vi "R vs T measurement - SImple.vi"() -> ()   [LabVIEW 2017]
uses:
  <vilib>/Utility/file.llb/Write Delimited Spreadsheet (DBL).vi
panel:
  in  "Tab Control":enum32{"Controlls"}(tab)
  in  "Source Meter address":refnum<visa-resource-name>="GPIB1::29::INSTR"
  out "Measured Resistance (Ohms)":dbl format="%#_6p"
  in  "Resistance Range Lower Limit (2 Ohm)":dbl=2.0 format="%#_6p"
  in  "Resistance Range Upper Limit (2E+8 Ohm)":dbl=200000000.0 format="%#_6p"
  in  "Resistance NPLC (0.1)":dbl=0.1
  in  "Resistance Range (2 Ohm)":dbl=2.0
  in  "Resistance Auto Range (T: Enable)":bool=TRUE
  in  "file to save data (dialog if empty)":path
  in  "Temperature controller Addres":refnum<visa-resource-name>
  in  "Input (0:A)":u16(ring) items=["A", "B", "C", "D"]
  out "Measured Temp (K)":dbl format="%.6p"
  in  "Record Rate (ms)":u32=1000
  in  "stop":bool
  in  "Error In":errorcluster
  # "Resistance vs Temperature Measurement"
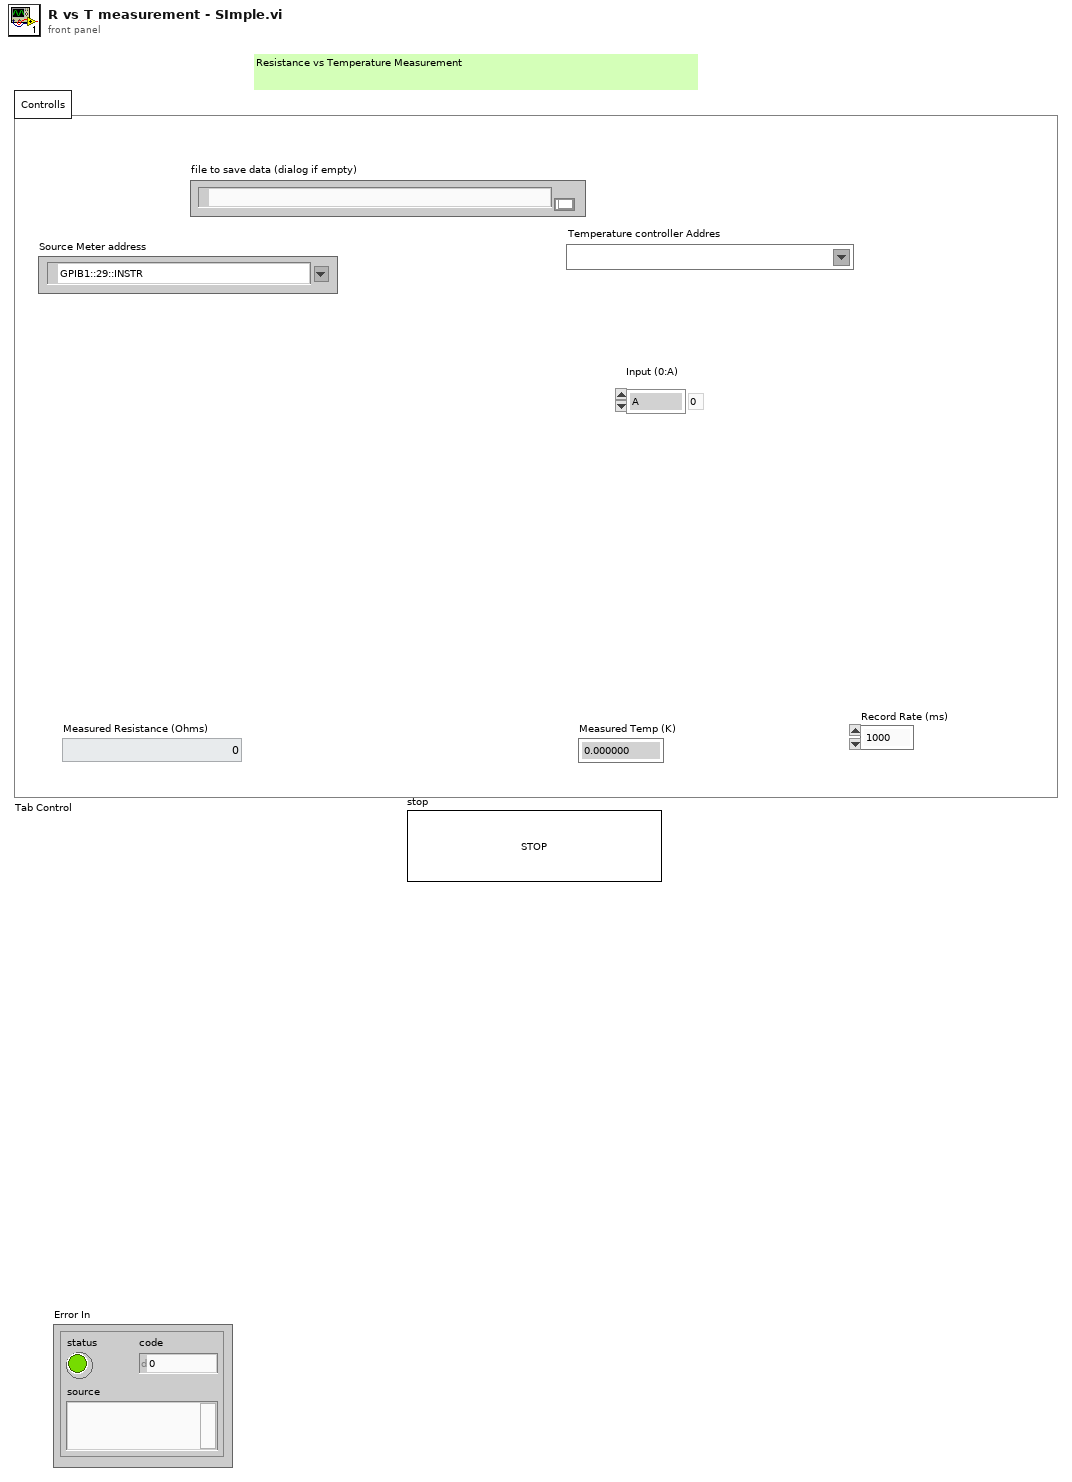
[diagram p1: front panel]
types:
  T1 = cluster{"Baud Rate":u32, "Parity":u16, "Data Bits":u16, "Stop Bits":u16, "Flow Control":u16}
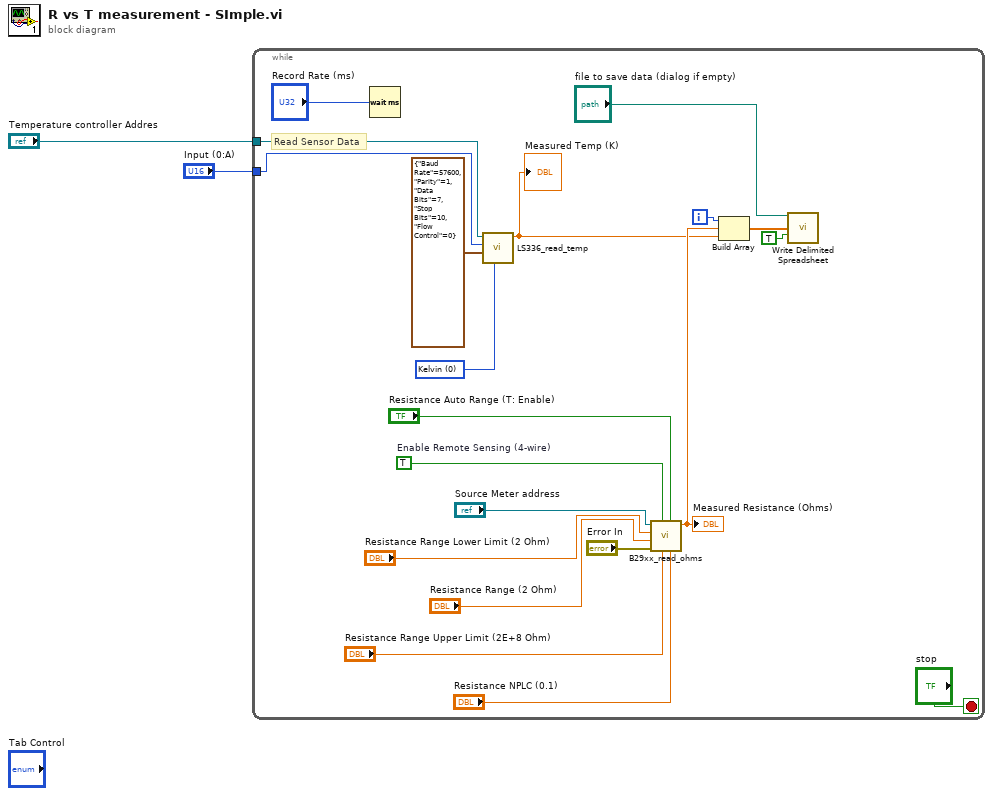
[diagram p0: block diagram]
diagram:
  n1 = while {
    tunnel: "Temperature controller Addres" -> [w9]
    tunnel: "Input (0:A)" -> [w8]
    i -> [w4]
    stop <- "stop" stop-if-true
    w10 = u16 0 items=["Kelvin", "Celsius", "Sensor Units"] ("Data Source (0:Kelvin)")
    w20 = TRUE  # Enable Remote Sensing (4-wire)
    # "Read Sensor Data"
    n2 = Wait (ms)(milliseconds to wait="Record Rate (ms)") -> ()  [unwired: 1 out]
    n3 = call "LS336_read_temp.vi"("Data Source (0:Kelvin)"=w10, "Serial Configuration"=T1 {"Baud Rate"=57600, "Parity"=1, "Data Bits"=7, "Stop Bits"=10, "Flow Control"=0}, "Input (0:A)"=w8, "VISA Refnum in"=w9) -> ("Sensor Data"=w3:dbl)  [unwired: 7 in]
    "Measured Temp (K)" <- w3
    n4 = call "B29xx_read_ohms.vi"("Resistance NPLC (0.1)"="Resistance NPLC (0.1)", "Resistance Auto Range (T: Enable)"="Resistance Auto Range (T: Enable)", "Resistance Range Upper Limit (2E+8 Ohm)"="Resistance Range Upper Limit (2E+8 Ohm)", "Enable Remote Sensing (4-wire)"=w20, "error in (no error)"="Error In", "Resistance Range (2 Ohm)"="Resistance Range (2 Ohm)", "Resistance Range Lower Limit (2 Ohm)"="Resistance Range Lower Limit (2 Ohm)", "VISA Refnum in"="Source Meter address") -> ("Measurement Result"=w14:dbl)  [unwired: 2 in, 1 out]
    "Measured Resistance (Ohms)" <- w14
    n5 = Build Array(w4, w14, w3) -> (w6:dbl[])
    n6 = call-poly <vilib>:"Write Delimited Spreadsheet.vi"("file path (dialog if empty)"="file to save data (dialog if empty)", "1D data"=w6, "append to file? (new file:F)"=TRUE) -> ()  [unwired: 11 in, 2 out]
  }
